vi "Pos Vel Accel.vi"(6 "distance/rotation":dbl=24.37875899 format="%#_13g", 10 "Starting pot value":dbl, 11 "PotDevRef":T1) -> (3 "Current Values":cluster{"pos":dbl, "vel":dbl, "accel":dbl})   [LabVIEW 2015]
uses:
  <vilib>/Rock Robotics/WPI/Potentiometer/WPI_PotentiometerDevRef.ctl
  <vilib>/Rock Robotics/SystemInterfaces/AI/FPGA_AIChannel.ctl
panel:
  in  "Limit":dbl=80.0 format="%#_13g"
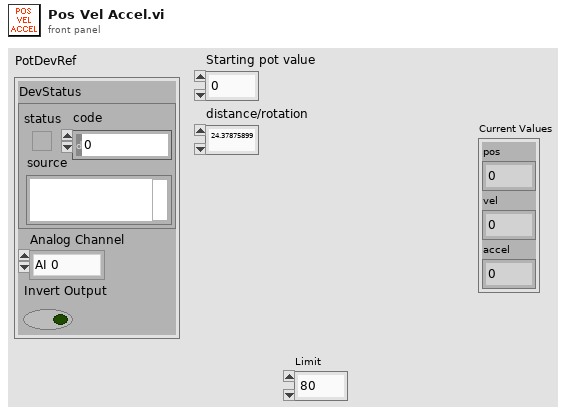
[diagram p1: front panel]
types:
  T1 = typedef "WPI_PotentiometerDevRef.ctl" = cluster{"DevStatus":errorcluster, "Analog Channel":T2, "Invert Output":bool}
  T2 = typedef "FPGA_AIChannel.ctl" = enum8{"AI 0", "AI 1", "AI 2", "AI 3", "AI MXP 0", "AI MXP 1", "AI MXP 2", "AI MXP 3", "Invalid"}
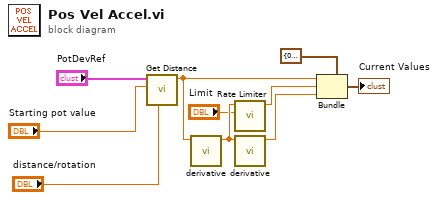
[diagram p0: block diagram]
diagram:
  n1 = call "Get Distance.vi"("distance/rotation"="distance/rotation", "Starting value"="Starting pot value", "PotDevRef"="PotDevRef") -> ("Distance"=w9:dbl)  [unwired: 8 in]
  n2 = call "derivative.vi"("x"=w9) -> ("dx/dt"=w2:dbl)  [unwired: 10 in]
  n3 = call "Rate Limiter.vi"("Limit"="Limit", "Value"=w2) -> ("Output"=w3:dbl)  [unwired: 9 in]
  n4 = call "derivative.vi"("x"=w2) -> ("dx/dt"=w10:dbl)  [unwired: 10 in]
  n5 = Bundle(cluster=cluster{"pos":dbl, "vel":dbl, "accel":dbl} {"pos"=0.0, "vel"=0.0, "accel"=0.0}, "pos"=w9, "vel"=w3, "accel"=w10) -> (→"Current Values":cluster{"pos":dbl, "vel":dbl, "accel":dbl})
